vi "Read Iterations Done.vi"(8 "error in (no error)":errorcluster, 11 "FWCS_ACS_Iterator in":refnum<class "FWCS_ACS_Iterator.lvclass">) -> (0 "error out":errorcluster, 2 "Iterations Done":u16, 3 "FWCS_ACS_Iterator out":refnum<class "FWCS_ACS_Iterator.lvclass">)   [LabVIEW 2018, in "FWCS_ACS_Iterator.lvclass"]
uses:
  FWCS_ACS_Iterator.lvclass
  FWCS_ACS_Iterator.lvclass/FWCS_ACS_Iterator.ctl
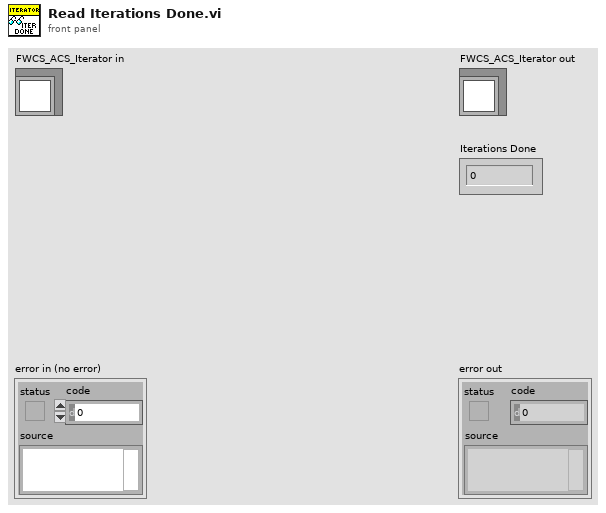
[diagram p1: front panel]
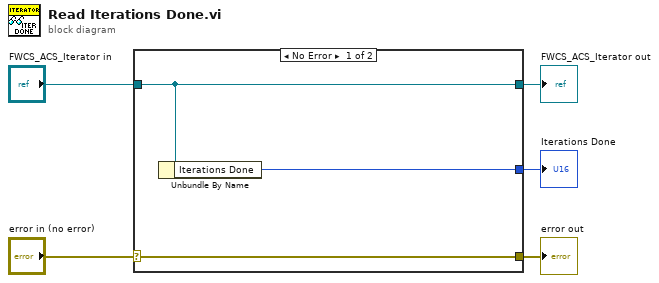
[diagram p0: block diagram]
diagram:
  n1 = case shown="No Error" "error in (no error)" {
    selector: "error in (no error)" -> [w8 w9]
    tunnel: [w8 w9] -> w4
    tunnel: [w7 w10] -> w2
    tunnel: "FWCS_ACS_Iterator in" -> [w7 w10]
    tunnel: [w6 _] -> w1
    frame No Error {
      n2 = Unbundle By Name(w7) -> ("Iterations Done"=w6:u16)
    }
    frame Error {
    }
  }
  "error out" <- w4
  "FWCS_ACS_Iterator out" <- w2
  "Iterations Done" <- w1
